vi "Query System Information Status.vi"(0 "VISA resource name":refnum<visa-resource-name>, 5 "System Information (0:Model)":i32(ring) items=["Model", "Type", "Serial Number", "System Time", "All"], 11 "error in (no error)":errorcluster) -> (4 "VISA resource name out":refnum<visa-resource-name>, 6 "Information Result String":string, 15 "error out":errorcluster)   [LabVIEW 2020, in "Anritsu Signal Analyzer Series.lvlib"]
doc: "Queries system information."
uses:
  Anritsu Signal Analyzer Series.lvlib
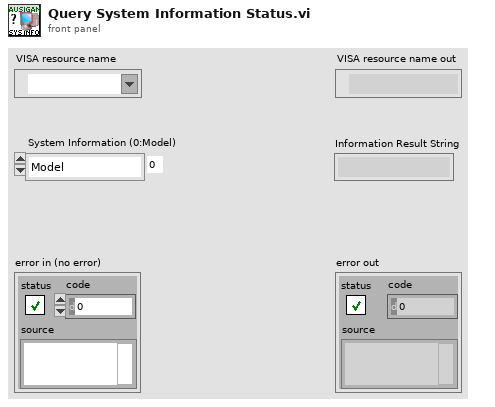
[diagram p1: front panel]
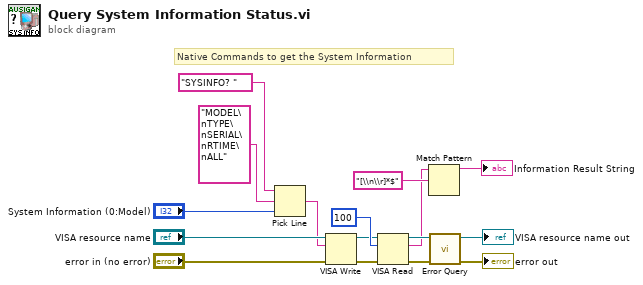
[diagram p0: block diagram]
diagram:
  # "Native Commands to get the System Information"
  n1 = Pick Line(string ("")="SYSINFO? " ("_Command"), multi-line string="MODEL\nTYPE\nSERIAL\nRTIME\nALL" ("文字列"), line index="System Information (0:Model)") -> (output string=w2:string)
  n2 = VISA Write(VISA resource name="VISA resource name", write buffer=w2, error in (no error)="error in (no error)") -> (VISA resource name out=w8:refnum<visa-resource-name>, error out=w9:errorcluster)  [unwired: 1 out]
  n3 = VISA Read(VISA resource name=w8, byte count=u32 100 ("byte count (0)"), error in (no error)=w9) -> (VISA resource name out=w6:refnum<visa-resource-name>, read buffer=w5:string, error out=w7:errorcluster)  [unwired: 1 out]
  n4 = Match Pattern(string=w5, regular expression="[\\n\\r]*$") -> (before substring=→"Information Result String":string)  [unwired: 1 in, 3 out]
  n5 = call "Error Query.vi"("error in (no error)"=w7, "VISA resource name"=w6) -> ("error out"=→"error out":errorcluster, "VISA resource name out"=→"VISA resource name out":refnum<visa-resource-name>)  [unwired: 6 in, 2 out]
